vi "Shooting Table.vi"() -> (3 "Chebyshev polynomials":cluster{"C":dbl[], "C":dbl[]})   [LabVIEW 2020]
panel:
  in  "degree":u16=2
  in  "Shooting Table":dbl[][](array[numeric])
  # "Distance, low, high"
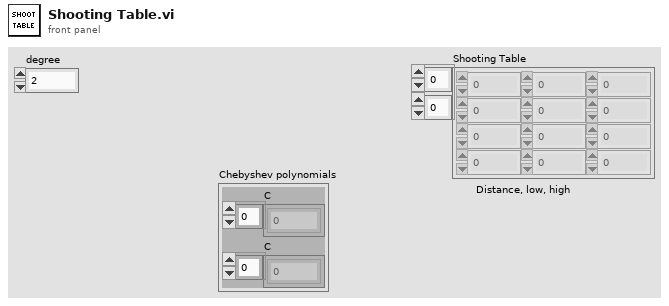
[diagram p1: front panel]
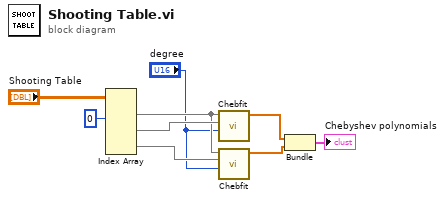
[diagram p0: block diagram]
diagram:
  n1 = Index Array(array="Shooting Table", index (col) #1=0 ("disabled index (col)")) -> (element #1=w6:dbl[], element #2=w7:dbl[], element #3=w5:dbl[])  [unwired: 5 in]
  n2 = call "Chebfit.vi"("degree"="degree", "Y"=w7, "X"=w6) -> ("C"=w3:dbl[])  [unwired: 8 in]
  n3 = call "Chebfit.vi"("degree"="degree", "Y"=w5, "X"=w6) -> ("C"=w2:dbl[])  [unwired: 8 in]
  n4 = Bundle("C"=w3, "C"=w2) -> (→"Chebyshev polynomials":cluster{"C":dbl[], "C":dbl[]})  [unwired: 1 in]
